vi "数据转换.vi"(11 "数据输入":string) -> (3 "波形数组":dbl[](array[numeric]))   [LabVIEW 2018]
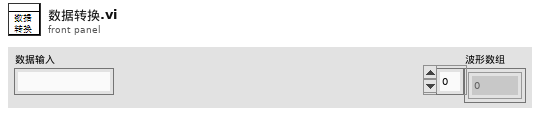
[diagram p1: front panel]
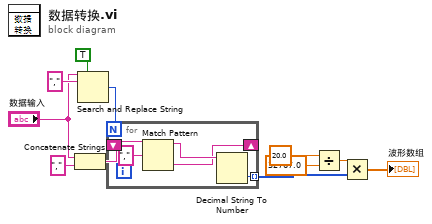
[diagram p0: block diagram]
diagram:
  n1 = Concatenate Strings("数据输入", "," ("字符串")) -> (w10:string)
  n2 = Search and Replace String(replace all?=TRUE ("替换全部？(F)"), input string="数据输入", search string="," ("搜索字符串")) -> (number of replacements=w8:i32)  [unwired: 5 in, 3 out]
  n3 = for {
    N: w8 -> [_]
    shift-right: [w13] -> _
    shift-left: w10 -> [w16]
    tunnel: [w12] -> w3 mode=indexing
    n4 = Match Pattern(string=w16, regular expression="," ("正则表达式")) -> (before substring=w14:string, after substring=w13:string)  [unwired: 1 in, 2 out]
    n5 = Decimal String To Number(string=w14) -> (number=w12:i32)  [unwired: 2 in, 1 out]
  }
  n6 = Divide(x=20.0, y=32767.0) -> (x/y=w4:dbl)
  n7 = Multiply(x=w4, y=w3) -> (x*y=→"波形数组":dbl[])
